vi "Check_and_Update_Coreset_Params.vi"(6 "NNPC_out":T3={"Name"="", "NN"={"Name"="", "No of Layers"=0, "mBatch"=1, "Layers"=[], "Dimty"=enum."In3D_Out3D", "Dims_In"={"C"=-1, "H"=-1, "W"=-1}, "Dims_Out"={"C"=-1, "H"=-1, "W"=-1}, "Working_Dir"=path "", "Train?"=FALSE, "Train_Params"={"Optimizer"=enum."SGD", "Beta_1"=0.999, "Beta_2"=0.999, "Weight Decay(L1)"=0.0, "Weight Decay(L2)"=0.0, "Data_Sampling"=enum."Random"}, "LR_Update_Policy"={"Policy_Type"=enum."Manual", "LR0"=0.0, "k"=0.0, "WarmUp_Policy"=enum."Step", "WarmUp_Iter"=100, "WarmUp_Ratio"=10.0}, "Session Data"={"Epochs"=0.0, "Tot_Iter"=1, "LR"=0.0, "LR_iter"=1}, "Ground_truth"={"Y"=variant}, "NNg_hdls"={"cudnn"=0, "cublas"=0, "stream"=0, "curand"=0}, "NN_Device"=enum."GPU", "GPU Id"=0, "Labels"=[], "Loss_Type"=enum."MSE", "Loss_Cfg_Prms"=variant, "NNG_WS"={"NNG_WS_Mem"=refnum, "Max_WS_Size"=-1}, "DryRun?"=FALSE}, "MemBank_Data"={"MemBank"=variant, "MemBank Norm"=variant}} {"NN"."LR_Update_Policy"."WarmUp_Ratio" min=1; "NN"."LR_Update_Policy"."WarmUp_Iter" min=1; "NN"."LR_Update_Policy"."LR0" format="%.7f"}, 7 "DS_Size":i32, 10 "Online_Coreset_Params in":T1={"Distance_Metric"=enum."Euclidean", "CoreSet_Size"=-1.0, "Start_idx"=3}, 11 "Coreset_Params in":T1={"Distance_Metric"=enum."Euclidean", "CoreSet_Size"=1.0, "Start_idx"=3} {"CoreSet_Size" format="%.3f"}) -> (2 "Online_Coreset_Params out":T1={"Distance_Metric"=enum."Euclidean", "CoreSet_Size"=0.0, "Start_idx"=3}, 3 "Coreset_Params out":T1={"Distance_Metric"=enum."Euclidean", "CoreSet_Size"=0.0, "Start_idx"=3})   [LabVIEW 2020]
uses:
  <vilib>/Ngene/DeepLTK Anomaly Detection Addon/Toolkit/API/Controls/NNPC_Coreset_Params.ctl
  <vilib>/Ngene/DeepLTK Anomaly Detection Addon/Toolkit/API/Controls/Distance_Metric.ctl
  <vilib>/Ngene/DeepLTK Anomaly Detection Addon/Toolkit/API/Controls/NNPC_Instance.ctl
  <vilib>/Ngene/Deep Learning Toolkit/Toolkit/NN_Network/Controls/NN.ctl
  <vilib>/Ngene/Deep Learning Toolkit/Toolkit/NN_Layers/Controls/NN_Layer_ref.ctl
  <vilib>/Ngene/Deep Learning Toolkit/Toolkit/NN_Network/Controls/NN_In_Out_Dim-ty.ctl
  <vilib>/Ngene/Deep Learning Toolkit/Toolkit/NN_Data/API/NN_Dims(C,H,W).ctl
  <vilib>/Ngene/Deep Learning Toolkit/Toolkit/NN_Train/Controls/NN_Train_Params.ctl
  <vilib>/Ngene/Deep Learning Toolkit/Toolkit/NN_Train/Controls/NN_Train_Optimizer.ctl
  <vilib>/Ngene/Deep Learning Toolkit/Toolkit/NN_Train/Controls/NN_Train_Data_Sampling.ctl
  <vilib>/Ngene/Deep Learning Toolkit/Toolkit/NN_Train/Controls/NN_LR_Policy_Cfg.ctl
  <vilib>/Ngene/Deep Learning Toolkit/Toolkit/NN_Train/Controls/NN_LR_Policy_Type.ctl
  <vilib>/Ngene/Deep Learning Toolkit/Toolkit/NN_Train/Controls/NN_Train_Session_Data.ctl
  <vilib>/Ngene/Deep Learning Toolkit/Toolkit/NN_Data/Controls/NN_Ground_truth.ctl
  <vilib>/Ngene/Deep Learning Toolkit/Toolkit/NNg/cuda/Controls/nng_cuda_handles.ctl
  <vilib>/Ngene/Deep Learning Toolkit/Toolkit/NN_Network/Controls/NN_Device.ctl
  <vilib>/Ngene/Deep Learning Toolkit/Toolkit/NN_Train/Controls/NN_Loss_Type.ctl
  <vilib>/Ngene/Deep Learning Toolkit/Toolkit/NNg/Network/WS/Controls/NNG_WS.ctl
  <vilib>/Ngene/Deep Learning Toolkit/Toolkit/NNg/Network/WS/Controls/NNg_WS_Mem_DVR.ctl
  <vilib>/Ngene/Deep Learning Toolkit/Toolkit/NNg/cuda/Controls/cuda_Mem_desc.ctl
  <vilib>/Ngene/DeepLTK Anomaly Detection Addon/Toolkit/API/Controls/MemBank_and_Norm_Variants.ctl
  <vilib>/Ngene/DeepLTK Anomaly Detection Addon/Toolkit/DeepLTK_Anomaly_Detection_Addon.lvlib
  <vilib>/Ngene/Deep Learning Toolkit/Toolkit/Deep_Learning_Toolkit_by_Ngene.lvlib
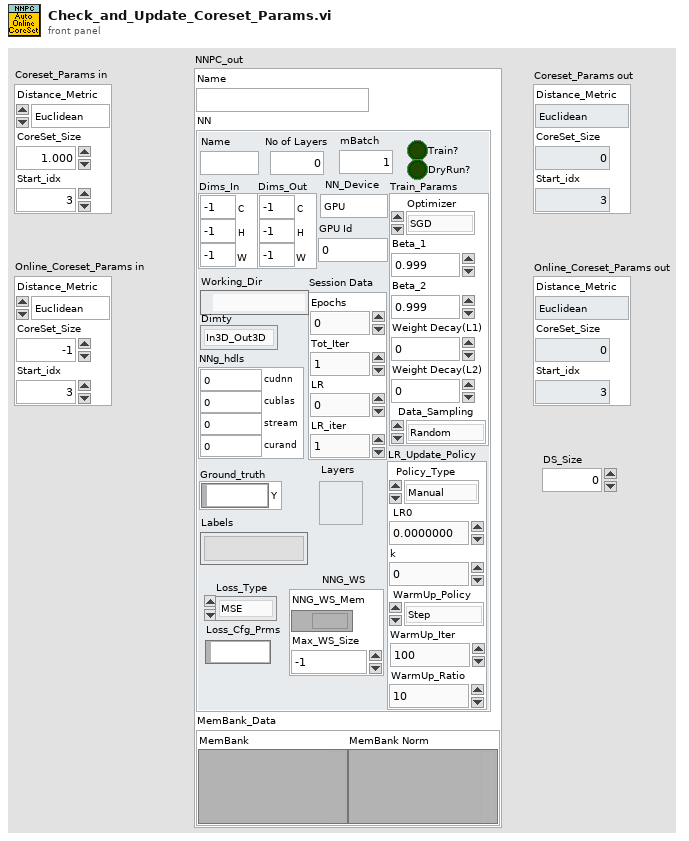
[diagram p1: front panel]
types:
  T1 = typedef "DeepLTK_Anomaly_Detection_Addon.lvlib/NNPC_Coreset_Params.ctl" = cluster{"Distance_Metric":T2, "CoreSet_Size":sgl, "Start_idx":i32}
  T2 = typedef "DeepLTK_Anomaly_Detection_Addon.lvlib/Distance_Metric.ctl" = enum16{"Euclidean", "Cosine"}
  T3 = typedef "DeepLTK_Anomaly_Detection_Addon.lvlib/NNPC_Instance.ctl" = cluster{"Name":string, "NN":T4, "MemBank_Data":T20}
  T4 = typedef "Deep_Learning_Toolkit_by_Ngene.lvlib/NN.ctl" = cluster{"Name":string, "No of Layers":i32, "mBatch":i32, "Layers":T5[], "Dimty":T6, "Dims_In":T7, "Dims_Out":T7, "Working_Dir":path, "Train?":bool, "Train_Params":T8, "LR_Update_Policy":T11, "Session Data":T13, "Ground_truth":T14, "NNg_hdls":T15, "NN_Device":T16, "GPU Id":i32, "Labels":string[], "Loss_Type":T17, "Loss_Cfg_Prms":variant, "NNG_WS":T18, "DryRun?":bool}
  T5 = typedef "Deep_Learning_Toolkit_by_Ngene.lvlib/NN_Layer_ref.ctl" = refnum<file>
  T6 = typedef "Deep_Learning_Toolkit_by_Ngene.lvlib/NN_In_Out_Dim-ty.ctl" = enum8{"In1D_Out1D", "In3D_Out1D", "In3D_Out3D", "In3D_OutBBox"}
  T7 = typedef "Deep_Learning_Toolkit_by_Ngene.lvlib/NN_Dims(C,H,W).ctl" = cluster{"C":i32, "H":i32, "W":i32}
  T8 = typedef "Deep_Learning_Toolkit_by_Ngene.lvlib/NN_Train_Params.ctl" = cluster{"Optimizer":T9, "Beta_1":sgl, "Beta_2":sgl, "Weight Decay(L1)":sgl, "Weight Decay(L2)":sgl, "Data_Sampling":T10}
  T9 = typedef "Deep_Learning_Toolkit_by_Ngene.lvlib/NN_Train_Optimizer.ctl" = enum16{"SGD", "Adam", "Adagrad", "Adadelta", "RMSProp", "Nesterov"}
  T10 = typedef "Deep_Learning_Toolkit_by_Ngene.lvlib/NN_Train_Data_Sampling.ctl" = enum16{"Random", "Sequential"}
  T11 = typedef "Deep_Learning_Toolkit_by_Ngene.lvlib/NN_LR_Policy_Cfg.ctl" = cluster{"Policy_Type":T12, "LR0":dbl, "k":sgl, "WarmUp_Policy":enum16{"Step", "Ramp"}, "WarmUp_Iter":i32, "WarmUp_Ratio":sgl}
  T12 = typedef "Deep_Learning_Toolkit_by_Ngene.lvlib/NN_LR_Policy_Type.ctl" = enum16{"Manual", "Step", "Exp", "1/t"}
  T13 = typedef "Deep_Learning_Toolkit_by_Ngene.lvlib/NN_Train_Session_Data.ctl" = cluster{"Epochs":sgl, "Tot_Iter":i32, "LR":sgl, "LR_iter":i32}
  T14 = typedef "Deep_Learning_Toolkit_by_Ngene.lvlib/NN_Ground_truth.ctl" = cluster{"Y":variant}
  T15 = typedef "Deep_Learning_Toolkit_by_Ngene.lvlib/nng_cuda_handles.ctl" = cluster{"cudnn":u64, "cublas":u64, "stream":u64, "curand":u64}
  T16 = typedef "Deep_Learning_Toolkit_by_Ngene.lvlib/NN_Device.ctl" = enum16{"CPU", "GPU"}
  T17 = typedef "Deep_Learning_Toolkit_by_Ngene.lvlib/NN_Loss_Type.ctl" = enum16{"None", "MSE", "CrossEntropy", "YOLO_v2", "YOLO_v4"}
  T18 = typedef "Deep_Learning_Toolkit_by_Ngene.lvlib/NNG_WS.ctl" = cluster{"NNG_WS_Mem":T19, "Max_WS_Size":i64}
  T19 = typedef "Deep_Learning_Toolkit_by_Ngene.lvlib/NNg_WS_Mem_DVR.ctl" = refnum<data-value>
  T20 = typedef "DeepLTK_Anomaly_Detection_Addon.lvlib/MemBank_and_Norm_Variants.ctl" = cluster{"MemBank":variant, "MemBank Norm":variant}
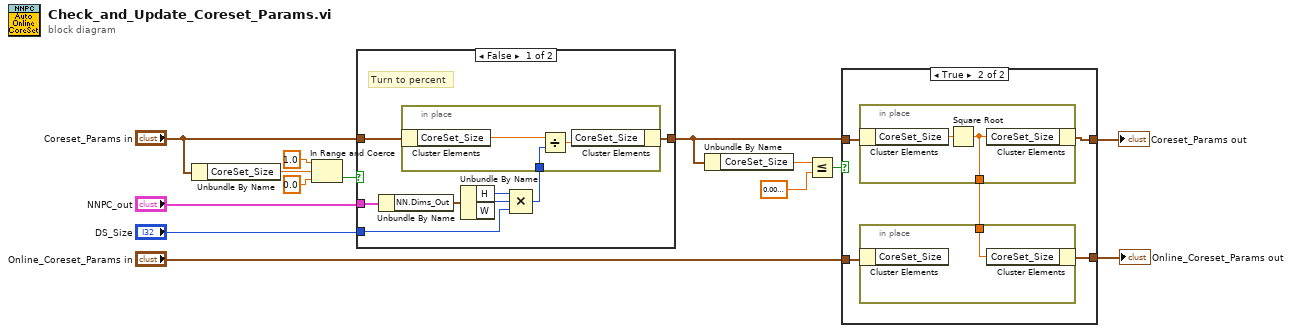
[diagram p0: block diagram]
diagram:
  n1 = Unbundle By Name("Coreset_Params in") -> ("CoreSet_Size"=w12:sgl)
  n2 = In Range and Coerce(upper limit=sgl 1.0, x=w12, lower limit=sgl 0.0) -> (In Range?=w9:bool)  [unwired: 1 out]
  n3 = case shown="False" w9 {
    tunnel: "Coreset_Params in" -> [w22 w26]
    tunnel: [w21 w26] -> w8
    tunnel: "NNPC_out" -> [w20 _]
    tunnel: "DS_Size" -> [w16 _]
    frame False {
      # "Turn to percent"
      n4 = Unbundle By Name(w20) -> ("NN.Dims_Out"=w19:T7)
      n5 = Unbundle By Name(w19) -> ("H"=w18:i32, "W"=w17:i32)
      n6 = Compound Arithmetic op=MULTIPLY(w18, w17, w16) -> (w15:i32)
      n7 = in-place {
        in-place-border: w15 -> [w23]
        n8 = in-place-cluster #1(w22) -> ("CoreSet_Size"=w25:sgl)
        n9 = Divide(x=w25, y=w23) -> (x/y=w24:sgl)
        n10 = in-place-cluster #1("CoreSet_Size"=w24) -> (w21:T1)
      }
    }
    frame True {
      # "in percent"
    }
  }
  n11 = Unbundle By Name(w8) -> ("CoreSet_Size"=w5:sgl)
  n12 = Less Or Equal?(x=w5, y=sgl 0.01) -> (x <= y?=w6:bool)
  n13 = case shown="True" w6 {
    tunnel: w8 -> [w28 w33]
    tunnel: "Online_Coreset_Params in" -> [w27 w32]
    tunnel: [w28 w30] -> w11
    tunnel: [w27 w29] -> w10
    frame False {
    }
    frame True {
      n14 = in-place {
        in-place-border: [w35] -> w31
        n15 = in-place-cluster #2(w33) -> ("CoreSet_Size"=w36:sgl)
        n16 = Square Root(x=w36) -> (sqrt(x)=w35:sgl)
        n17 = in-place-cluster #2("CoreSet_Size"=w35) -> (w30:T1)
      }
      n18 = in-place {
        in-place-border: w31 -> [w34]
        n19 = in-place-cluster #3(w32) -> ()  [unwired: 1 out]
        n20 = in-place-cluster #3("CoreSet_Size"=w34) -> (w29:T1)
      }
    }
  }
  "Coreset_Params out" <- w11
  "Online_Coreset_Params out" <- w10
